vi "closeSWWindows.vi"(8 "error in (no error)":errorcluster) -> (0 "error out":errorcluster)   [LabVIEW 2012]
uses:
  user32.dll
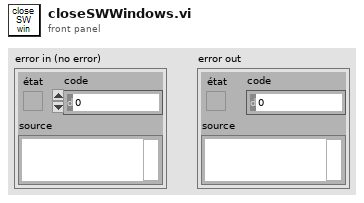
[diagram p1: front panel]
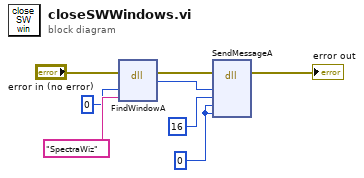
[diagram p0: block diagram]
diagram:
  w7 = u32 0 ("lParam")
  n1 = dll-call lib="user32.dll" fn="FindWindowA" label="FindWindow"(error in="error in (no error)", "lpszClassName"=0, "lpszWindowName"="SpectraWiz") -> (error out=w4:errorcluster, "hWnd"=w5:u32)  [unwired: 4 in, 1 out]
  n2 = dll-call lib="user32.dll" fn="SendMessageA" label="SendMessage"(error in=w4, "hWnd"=w5, "uMsg"=u32 16, "wParam"=w7, "lParam"=w7) -> (error out=→"error out":errorcluster)  [unwired: 7 in, 1 out]
